vi "Cluster Ref.vi"(8 "error out":errorcluster, 9 "Label Text":string, 10 "Input Array":string[](array[string]), 11 "Cluster Reference":refnum<vi>) -> (2 "Array Out":string[](array[string]), 3 "Controls[]":refnum<vi>[](array[refnum]))   [LabVIEW 2021]
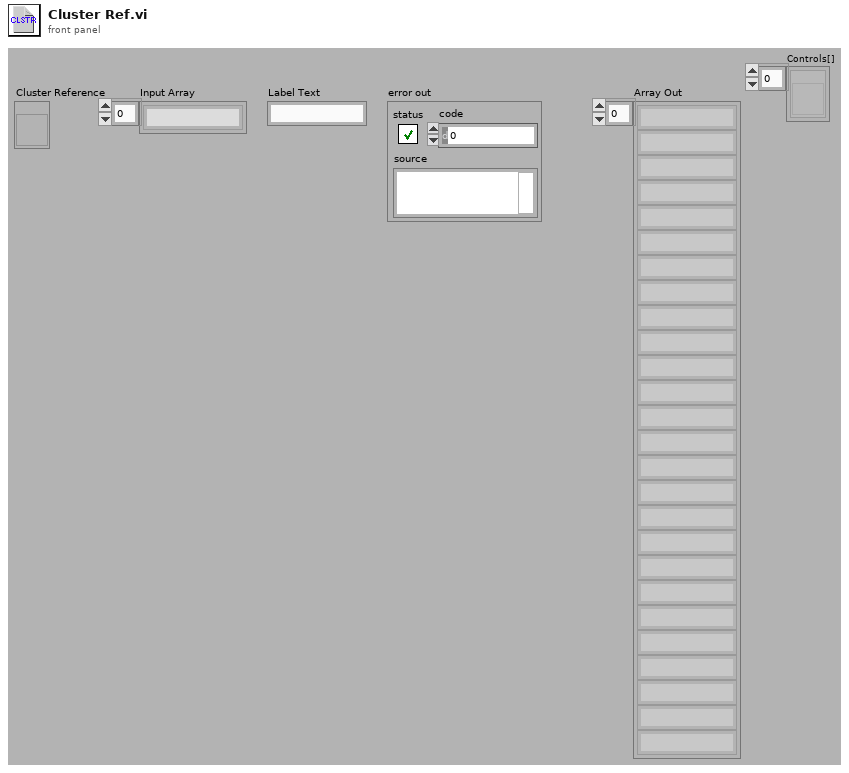
[diagram p1: front panel]
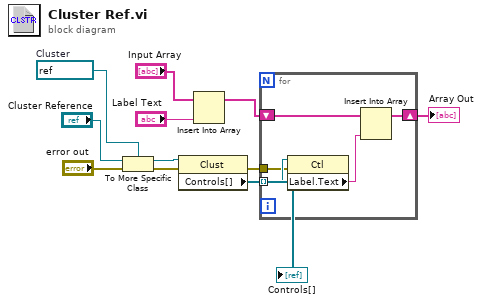
[diagram p0: block diagram]
diagram:
  w5 = refnum<vi> refnum  # Cluster
  n1 = To More Specific Class(target class=w5, reference="Cluster Reference", error in="error out") -> (specific class reference=w3:refnum<vi>, error out=w1:errorcluster)
  n2 = property class="Clust"(reference=w3, error in=w1) -> (error out=w10:errorcluster, "Controls[]"=w6:refnum<vi>[])  [unwired: 1 out]
  "Controls[]" <- w6
  n3 = Insert Into Array(array="Input Array", new element="Label Text") -> (w8:string[])  [unwired: 1 in]
  n4 = for {
    tunnel: w6 -> [w16] mode=indexing
    shift-right: [w12] -> w9
    shift-left: w8 -> [w15]
    tunnel: w10 -> [w14]
    n5 = property class="Ctl"(reference=w16, error in=w14) -> ("Label.Text"=w13:string)  [unwired: 2 out]
    n6 = Insert Into Array(array=w15, new element=w13) -> (w12:string[])  [unwired: 1 in]
  }
  "Array Out" <- w9
